vi "SeqUpdateNewTables.vi"(8 "error in (no error)":errorcluster, 11 "List_UI in":refnum<class "List_UI.lvclass">) -> (0 "error out":errorcluster, 3 "List_UI out":refnum<class "List_UI.lvclass">)   [LabVIEW 2015, in "List_UI.lvclass"]
uses:
  List_UI.lvclass
panel:
  in  "Delta":i32
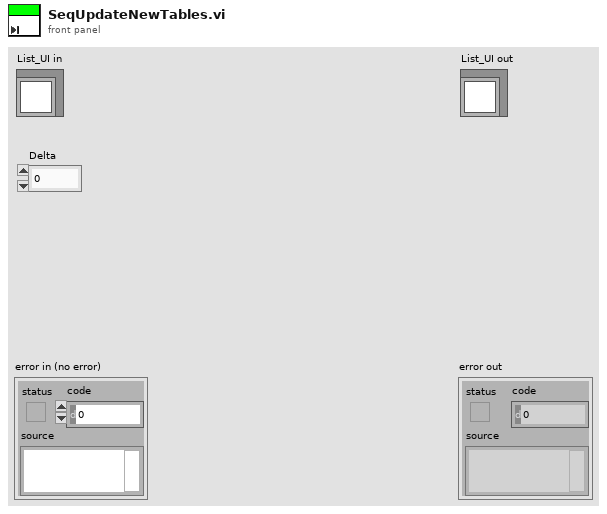
[diagram p1: front panel]
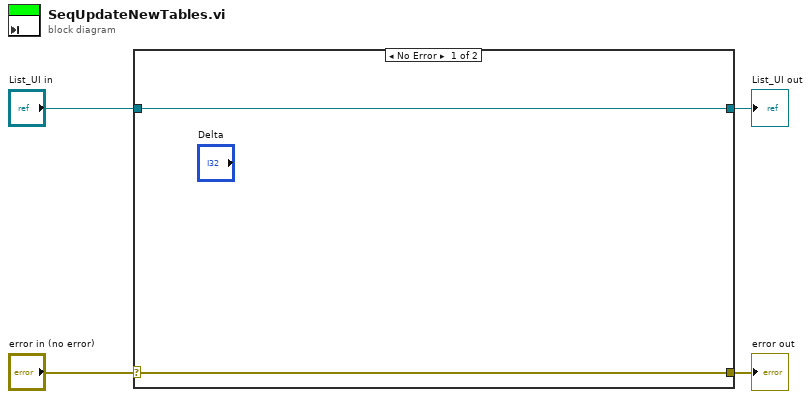
[diagram p0: block diagram]
diagram:
  n1 = case shown="No Error" "error in (no error)" {
    selector: "error in (no error)" -> [w5 w8]
    tunnel: [w5 w8] -> w3
    tunnel: [w6 w7] -> w1
    tunnel: "List_UI in" -> [w6 w7]
    frame No Error {
    }
    frame Error {
    }
  }
  "error out" <- w3
  "List_UI out" <- w1
